vi "getStatusMoving.vi"(8 "error in":errorcluster, 9 "status moving in":bool=TRUE, 10 "axis in":u8, 11 "connection ID":refnum<k5>) -> (0 "error out":errorcluster, 1 "status moving out":bool=TRUE, 2 "axis out":u8, 3 "connection ID":refnum<k5>)   [LabVIEW 2019]
panel:
  in  "Get Command":string="com.attocube.amc.status.getStatusMoving"
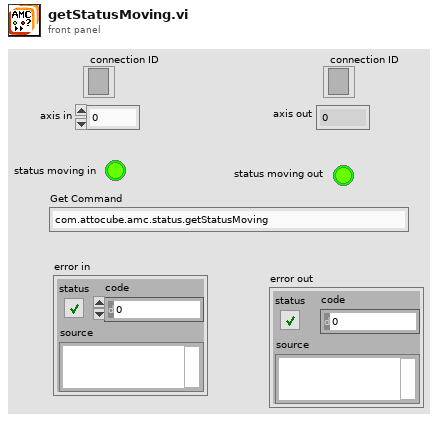
[diagram p1: front panel]
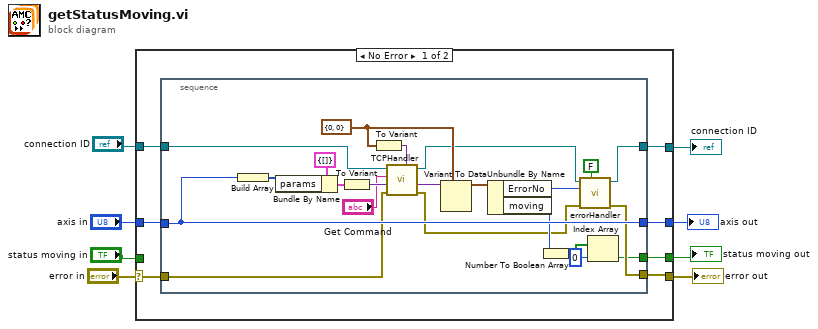
[diagram p0: block diagram]
diagram:
  n1 = case shown="No Error" "error in" {
    selector: "error in" -> [w9 w39]
    tunnel: "axis in" -> [w15 w41]
    tunnel: [w10 w39] -> w7
    tunnel: [w12 w41] -> w6
    tunnel: [w11 w40] -> w5
    tunnel: [w13 w38] -> w4
    tunnel: "connection ID" -> [w14 w38]
    tunnel: "status moving in" -> [_ w40]
    frame No Error {
      n2 = stacked-sequence {
        tunnel: [w19] -> w13
        tunnel: w14 -> [w27]
        tunnel: w15 -> [w29]
        tunnel: [w29] -> w12
        tunnel: [w28] -> w10
        tunnel: [w21] -> w11
        tunnel: w9 -> [w17]
        frame #0 {
          w25 = cluster{"ErrorNo":i32, "moving":i64} {"ErrorNo"=0, "moving"=0} ("input cluster")
          n3 = Build Array(w29) -> (w33:u8[])
          n4 = Bundle By Name(cluster=cluster{"params":i32[]} {"params"=[]} ("input cluster"), "params"=w33) -> (w34:cluster{"params":i32[]})
          n5 = To Variant(anything=w34) -> (Variant=w35:variant)
          n6 = To Variant(anything=w25) -> (Variant=w26:variant)
          n7 = call <userlib>:"TCPHandler.vi"("result Types"=w26, "error in (no error)"=w17, "params"=w35, "method"="Get Command", "connection ID"=w27) -> ("error out"=w16:errorcluster, "result"=w31:variant, "connection ID"=w20:refnum<k5>)  [unwired: 3 in, 1 out]
          n8 = Variant To Data(type=w25, Variant=w31) -> (data=w36:cluster{"ErrorNo":i32, "moving":i64})  [unwired: 1 in, 1 out]
          n9 = Unbundle By Name(w36) -> ("ErrorNo"=w37:i32, "moving"=w22:i64)
          n10 = Number To Boolean Array(number=w22) -> (Boolean array=w23:bool[])
          n11 = call <userlib>:"errorHandler.vi"("show popup"=FALSE, "error in"=w16, "error number"=w37, "connection ID"=w20) -> ("error out"=w28:errorcluster, "connection ID"=w19:refnum<k5>)  [unwired: 6 in]
          n12 = Index Array(array=w23, index=0) -> (element=w21:bool)
        }
      }
    }
    frame Error {
    }
  }
  "error out" <- w7
  "axis out" <- w6
  "status moving out" <- w5
  "connection ID" <- w4
